vi "Robot Global Data.vi"() -> ()   [LabVIEW 2015]
doc: "This global VI can contain as many global variables as you need. Place a control on the panel, give it a good name. To read or write to it from a VI, drag the icon to the diagram of that VI. You can also drag from the project. Click on the node to change which global you access. You shouldn't have multiple locations writing to a global or it will cause a race-condition."
uses:
  <vilib>/Rock Robotics/WPI/DriverStation/WPI_DriverStationRobotMode2.ctl
  <vilib>/Rock Robotics/WPI/CAN/TalonSRX/WPI_CANTalonSRX_APIControlMode.ctl
  <vilib>/Rock Robotics/WPI/Solenoid/WPI_SolenoidValue.ctl
  <vilib>/Rock Robotics/WPI/Camera/WPI_CameraImageSize.ctl
panel:
  in  "Y Axis Offset":dbl
  in  "VisionShooterValue":dbl
  in  "SuperVisionEnabled":bool
  in  "VisionEncoderError":dbl
  in  "VisionEncoderTarget":dbl
  in  "VisionAfterOffset":dbl
  in  "ScalerArmMotorHasDeployed":bool
  in  "ScalerArmSolenoidHasDeployed":bool
  in  "LowBarWonderArmPosition":dbl
  in  "RollerTarget":dbl
  in  "RightDriveMotorSpeed":dbl
  in  "LeftDriveMotorSpeed":dbl
  in  "LoopTime":dbl
  in  "RightMotorOutput":dbl
  in  "LeftMotorOutput":dbl
  in  "LeftRightMotorInput":dbl
  in  "ForwardBackMotorInput":dbl
  out "ms to process":u32
  in  "PickupBallPosition":dbl
  in  "ShooterManualControl":dbl
  in  "VisionNavXError":dbl
  in  "MomentFactor":dbl
  in  "VisionGyroTarget":dbl
  in  "HighestAspect":dbl
  in  "image size":T1=enum."320x240"
  in  "VisionCurrentState":enum16{"Disabled", "Enable", "Suspended", "PID"}(ring)
  in  "HighGoalShootPosition":dbl
  in  "VisionCenterDistance":dbl
  out "ShooterState":T2(ring)=enum."Hold"
  in  "ActualRPM1":dbl
  in  "DesiredRPM1":dbl
  in  "AutoShooterSpeedValue":dbl
  in  "RightMotorInput":dbl
  in  "LeftMotorInput":dbl
  in  "DashboardRollerArmActual":dbl
  in  "DashboardRollerArmDesired":dbl
  in  "DashboardShooterAngleActual":dbl
  in  "DashboardShooterAngleDesired":dbl
  in  "RollerArmHeight":dbl
  in  "Wonder Arm Vision Position":dbl
  in  "ShooterMotorAmpsLeft":dbl
  in  "ShooterMotorAmpsRight":dbl
  in  "ShooterMotorRightActualRPM":dbl
  in  "ShooterMotorRightDesiredRPM":dbl
  in  "TeleopButtonScalerSolenoid":bool
  in  "BallHaloCylinder":T3
  in  "BallShooterCylinder":T3
  in  "NavXConnected":bool
  in  "Right Motor Encoder":dbl
  in  "Left Motor Encoder":dbl
  in  "ScalerArmCommand":dbl
  in  "AutoVisionControl":bool
  in  "Auto1FileStatus":string
  in  "Auto0CurrentFile":string
  in  "SuckSpeed":dbl
  in  "BumperShotSpeed":dbl
  in  "HighGoalSpeed":dbl
  in  "LowGoalSpeed":dbl
  in  "ShooterWheelCountsPerRevolution":dbl=80.0
  in  "TeleopButtonScaler":bool
  in  "AnalogGyroAngle":dbl
  in  "IsStalled":bool
  in  "ControllerRumble":bool
  in  "IsCompBot":bool
  in  "AutoShootCommand":bool
  in  "AutoShooterSpeedControl":bool
  in  "AutoShooterAngleSetHeight":dbl
  in  "AutoShooterArmAngleControl":bool
  in  "ScalerControl":dbl
  in  "TapeMeasureControl":dbl
  in  "SuckButton":bool
  in  "ShooterAngleOffset":dbl
  in  "AutoShoot":bool
  in  "ShootCommand":bool
  in  "IsInPosition":bool
  in  "Gyro180":dbl
  in  "DashboardRollerArmState":T4(ring)
  in  "DashboardShooterAngleState":T5(ring)
  in  "DashboardWheelTwoActual":dbl
  in  "DashboardWheelTwoDesired":dbl
  in  "DashboardWheelOneActual":dbl
  in  "DashboardWheelOneDesired":dbl
  in  "PhotoeyeBall":bool
  in  "AngleMotorState":T5(ring)=enum."ResetForward"
  in  "TeleopButtonAllUp":bool
  in  "AutoRollerArmHeight":dbl
  in  "AutoArmControl":bool
  in  "TeleopButtonLowBar":bool
  in  "RollerArmDownPosition":dbl
  in  "RollerArmUpPosition":dbl
  out "DriveStraightRampartsState":T6(ring)
  in  "NavXAcceleration":T7
  in  "NavXDisplacement":T8
  in  "TeleopButtonShooterAngle\nEmergencyManual":bool
  in  "TeleopButtonRollerAngle\nEmergencyManual":bool
  in  "ManualControlButton":bool
  in  "TeleopButtonRollerPickupBall":bool
  in  "TeleopButtonRollerDown":bool
  in  "TeleopButtonRollerUp":bool
  in  "TeleopInputRollerElevation":dbl
  in  "TeleopButtonAngleMotorReset":bool
  in  "IsLevel":bool
  out "NavXRotation":T9
  in  "ControlMode2":T10=enum."Speed"
  in  "ControlMode1":T10=enum."Speed"
  in  "TeleopButtonBumperShot":bool
  in  "Shooter Button":bool
  in  "TeleopButtonShooterAngleHighGoal":bool
  in  "Low Goal Shooter Button":bool
  in  "IsAutoTargeting":bool
  in  "IsHaloDrive":bool
  in  "GoalCentered":bool
  in  "Vision/Has Goal":bool
  out "Robot Mode":T11
  out "Detected Targets":T12(array[cluster]) {"Normalized Rect"."Numeric 5" format="%#_2g"; "Normalized Rect"."Numeric 3" format="%#_2g"; "Normalized Rect"."Numeric 2" format="%#_2g"; "Normalized Rect"."Numeric" format="%#_2g"}
  in  "Enable Vision":bool=TRUE
  # "Floats and Integers"
  # "Booleans"
  # "Teleop Inputs"
  # "Autonomous Inputs"
  # "Teleop Inputs"
  # "Autonomous Inputs"
  # "Bot Status"
  # "Roller Arm Constants"
  # "Shooter Wheel Constants"
  # "Enums"
  # "State Machines"
  # "Other"
  # "NavX and Gyro"
  # "Shooter Wheel"
  # "Other"
  # "Drive Train and Roller Arm and Shooter Arm"
  # "Vision and Other"
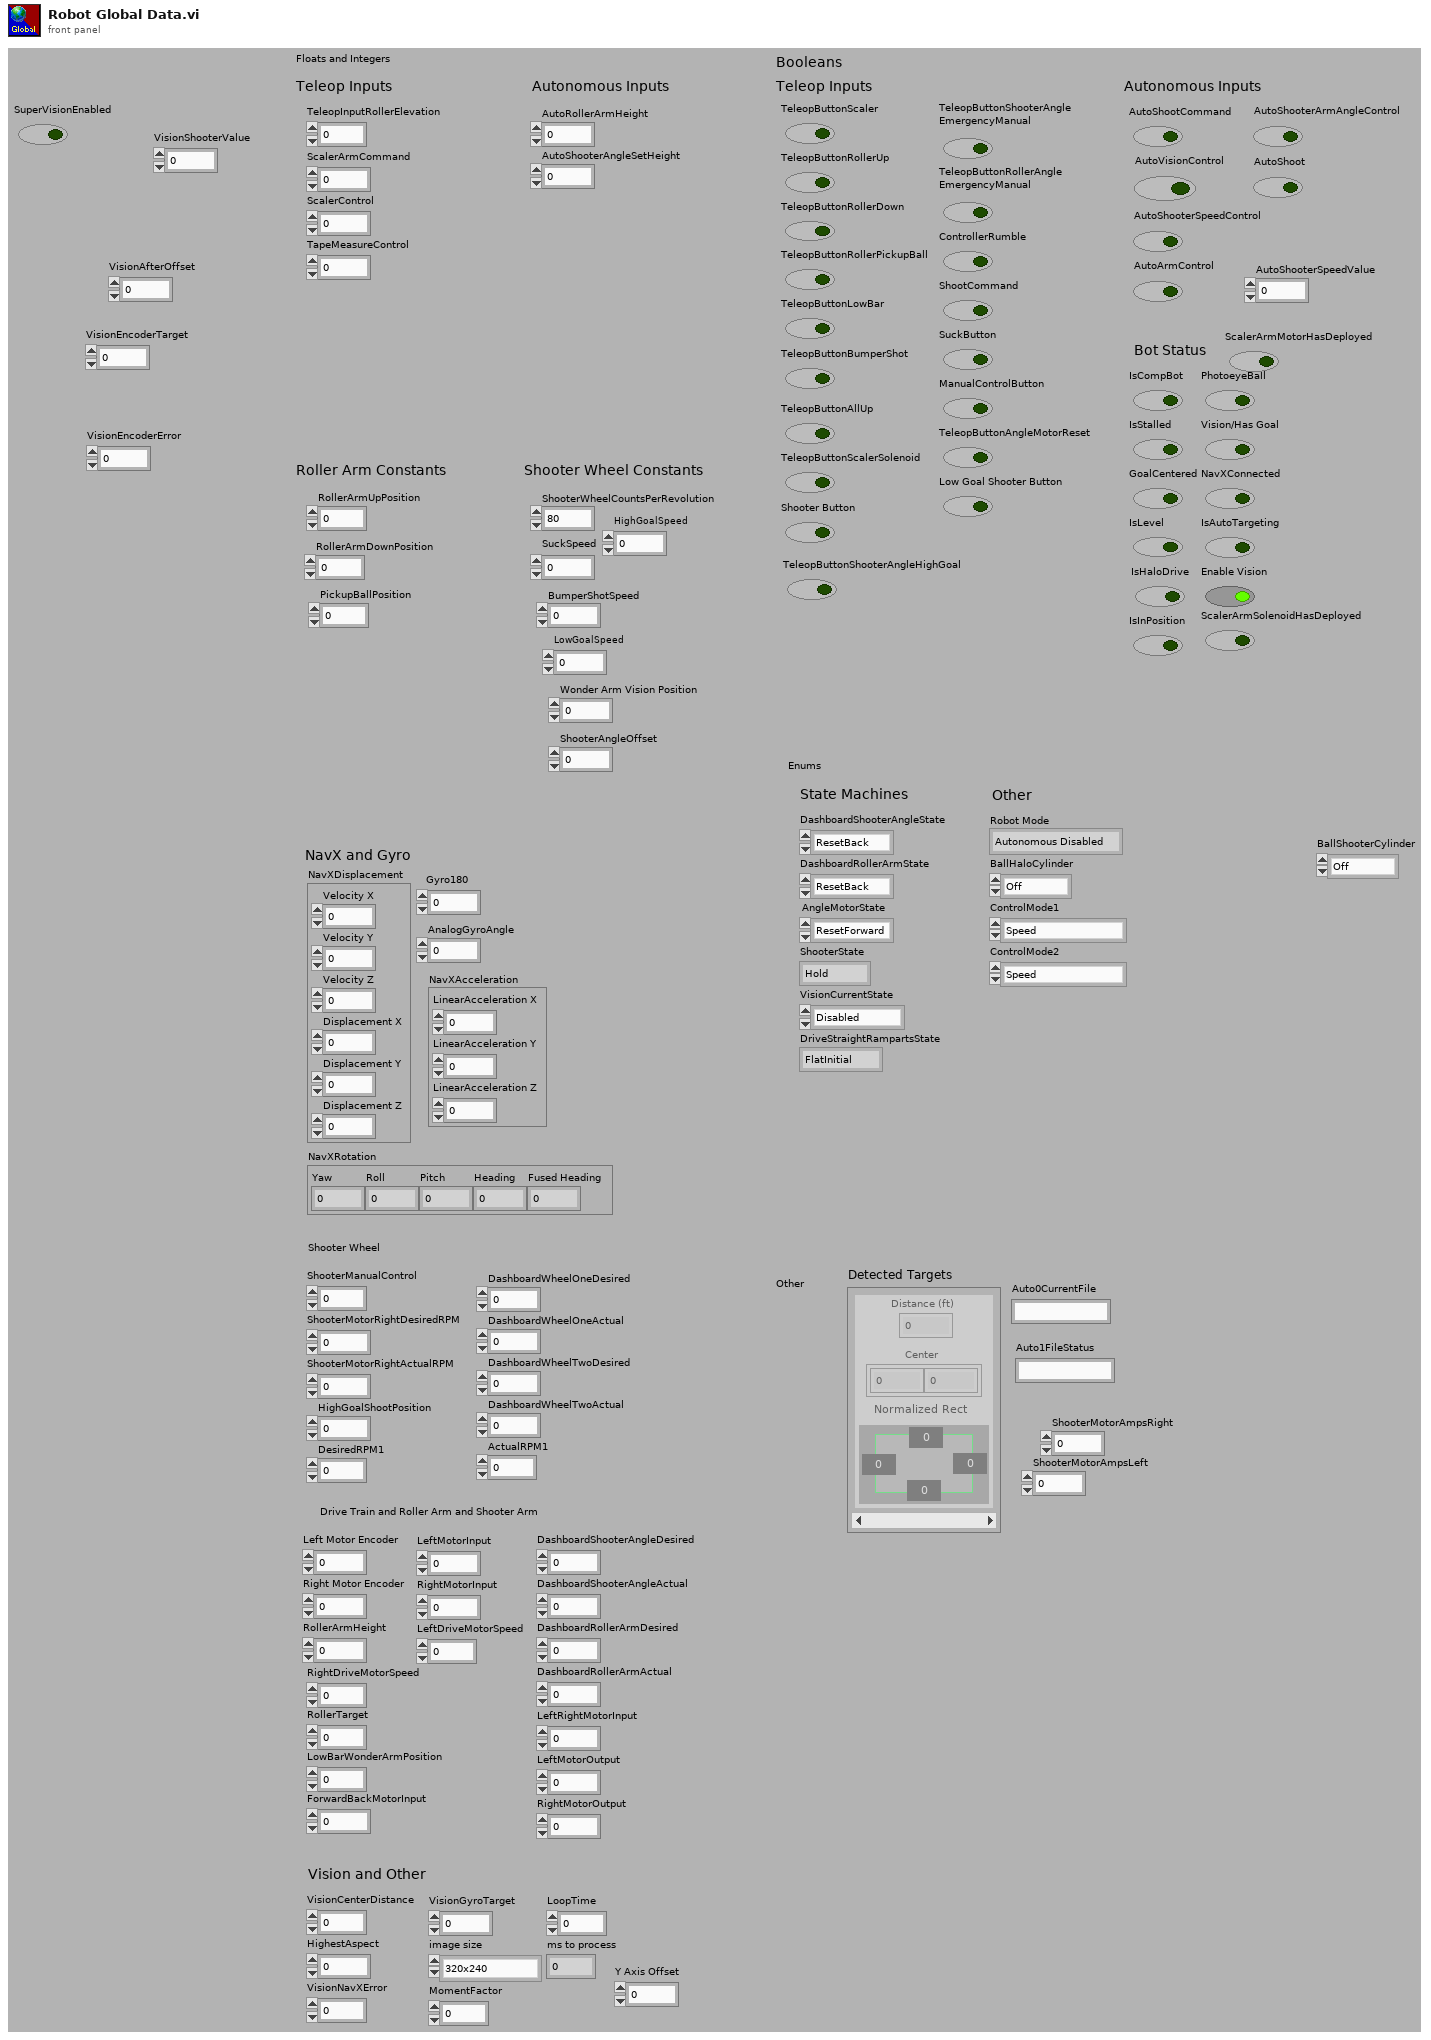
[diagram p1: front panel]
types:
  T1 = typedef "WPI_CameraImageSize.ctl" = enum16{"640x480", "320x240", "160x120", "Custom"}
  T2 = enum16{"Empty", "Suck", "Hold", "LowGoal", "HighGoal", "BumperShot", "Shoot", "Dwell"}
  T3 = typedef "WPI_SolenoidValue.ctl" = enum16{"Off", "On", "Forward", "Reverse"}
  T4 = enum16{"ResetBack", "EmergencyManualControl", "ResetForward", "Hold", "Reset", "ManualControl"}
  T5 = enum16{"ResetBack", "ResetForward", "Reset", "Hold", "HighGoal", "LowGoal", "BumperShot", "EmergencyManualControl"}
  T6 = enum16{"FlatInitial", "AngleUp", "AngleDown", "FlatFinal"}
  T7 = cluster{"LinearAcceleration X":dbl, "LinearAcceleration Y":dbl, "LinearAcceleration Z":dbl}
  T8 = cluster{"Velocity X":dbl, "Velocity Y":dbl, "Velocity Z":dbl, "Displacement X":dbl, "Displacement Y":dbl, "Displacement Z":dbl}
  T9 = cluster{"Yaw":dbl, "Roll":dbl, "Pitch":dbl, "Heading":dbl, "Fused Heading":dbl}
  T10 = typedef "WPI_CANTalonSRX_APIControlMode.ctl" = enum8{"Percent VBus", "Speed", "Position", "Slave", "Unchanged / Invalid", "Voltage Compensation", "Current", "Motion Profile"}
  T11 = typedef "WPI_DriverStationRobotMode2.ctl" = enum16{"Autonomous Disabled", "Autonomous Enabled", "Teleop Disabled", "Teleop Enabled", "Disconnected", "Finish", "Test Disabled", "Test Enabled", "Emergency Stopped"}
  T12 = cluster{"Distance (ft)":dbl, "Center":cluster{dbl, dbl}, "Normalized Rect":cluster{"Numeric":dbl, "Numeric 2":dbl, "Numeric 3":dbl, "Numeric 5":dbl}}[]
diagram:
